vi "Generate Arbitrary Mask.vi"() -> ()   [LabVIEW 2016]
uses:
  <vilib>/vision/NI_Vision_Development_Module.lvlib
panel:
  out "Image":T1(plugin-control)
  in  "Scale":dbl
  out "Intensity Graph":u8[][](graph)
  in  "Data":dbl[][](graph)=array180x1000[180000 elements]
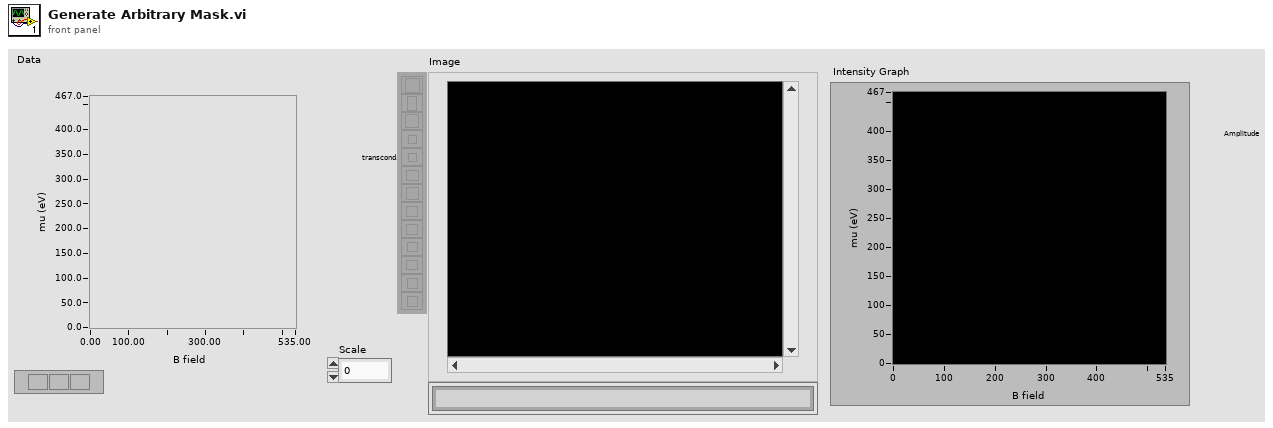
[diagram p1: front panel]
types:
  T1 = typedef "IMAQ Image.ctl" = refnum<image>
  T2 = typedef "Image Type" = u32
  T3 = cluster{"Global Rectangle":i32[], "Contours":cluster{"Contour Type":u32, "ROI Type":u32, "Points":i32[]}[]}
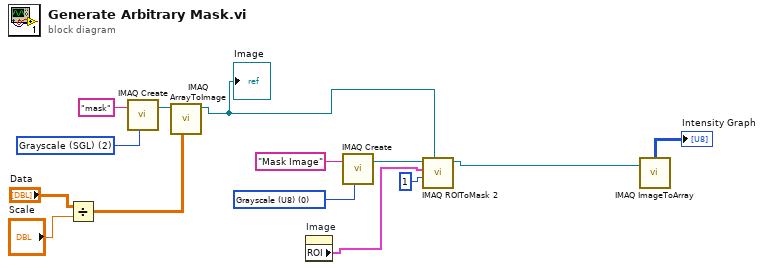
[diagram p0: block diagram]
diagram:
  w10 = T2 0 items=["Grayscale (U8)", "Grayscale (I16)", "Grayscale (SGL)", "Complex (CSG)", "RGB (U32)", "HSL (U32)", "RGB (U64)", "Grayscale (U16)"] ("Image Type")
  w13 = T2 2 items=["Grayscale (U8)", "Grayscale (I16)", "Grayscale (SGL)", "Complex (CSG)", "RGB (U32)", "HSL (U32)", "RGB (U64)", "Grayscale (U16)"] ("Image Type")
  n1 = Divide(x="Data", y="Scale") -> (x/y=w4:dbl[][])
  n2 = call "IMAQ Create"("Image Name"="mask", "Image Type"=w13) -> ("New Image"=w12:T1)  [unwired: 3 in, 1 out]
  n3 = call "IMAQ ArrayToImage"("Image Pixels (Float)"=w4, "Image"=w12) -> ("Image Out"=w2:T1)  [unwired: 8 in, 1 out]
  "Image" <- w2
  n4 = property on="Image" class="ImageControl"() -> ("ROI"=w1:T3)  [unwired: 2 in, 2 out]
  n5 = call "IMAQ Create"("Image Name"="Mask Image", "Image Type"=w10) -> ("New Image"=w9:T1)  [unwired: 3 in, 1 out]
  n6 = call "IMAQ ROIToMask 2"("Image Model"=w2, "Filling Value (255)"=1, "ROI Descriptor"=w1, "Image"=w9) -> ("Image Out"=w3:T1)  [unwired: 5 in, 2 out]
  n7 = call "IMAQ ImageToArray"("Image"=w3) -> ("Image Pixels (U8)"=→"Intensity Graph":u8[][])  [unwired: 3 in, 4 out]
